vi "Get PIM System Directory.vi"(7 "Relative Path":path, 11 "Directory":T1(ring)) -> (3 "PIM Path":path)   [LabVIEW 2011]
uses:
  <vilib>/Utility/sysdir.llb/System Directory Type.ctl
panel:
  in  "Base Directory (Kaelus)":enum16{"Kaelus", "Summitek"}(ring)
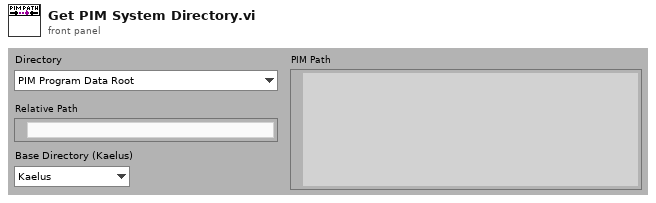
[diagram p1: front panel]
types:
  T1 = enum16{"PIM Program Data Root", "Instrument Calibration Files", "Instrument Configuration Files", "User Data", "User Configurations", "SI-90 Saved Calibrations"}
  T2 = typedef "System Directory Type.ctl" = i32
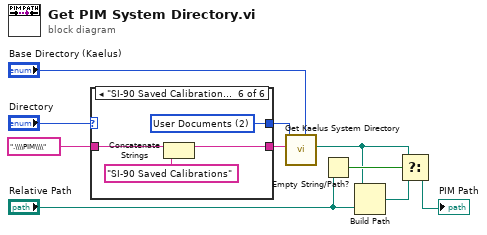
[diagram p0: block diagram]
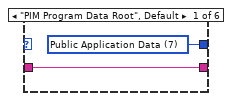
[diagram p2: hidden frame]
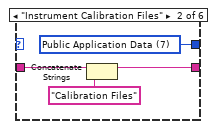
[diagram p3: hidden frame]
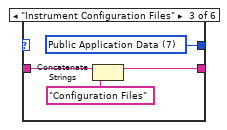
[diagram p4: hidden frame]
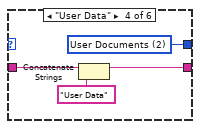
[diagram p5: hidden frame]
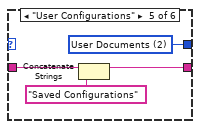
[diagram p6: hidden frame]
diagram:
  n1 = case shown="\"SI-90 Saved Calibrations\"" "Directory" {
    tunnel: ".\\\\PIM\\\\" ("Relative Application Path") -> [w12 w16 w20 w24 w28 w32]
    tunnel: [w12 w14 w18 w22 w26 w30] -> w8
    tunnel: [w11 w13 w17 w21 w25 w29] -> w2
    frame "PIM Program Data Root", Default {
      w11 = T2 7 items=["User Home", "User Desktop", "User Documents", "User Application Data", "User Preferences", "User Temporary", "Public Documents", "Public Application Data", "Public Preferences", "System Core Libraries", "System Installed Libraries", "Application Files", "Boot Volume Root"] ("Directory Type (Public App Data)")
    }
    frame "Instrument Calibration Files" {
      w13 = T2 7 items=["User Home", "User Desktop", "User Documents", "User Application Data", "User Preferences", "User Temporary", "Public Documents", "Public Application Data", "Public Preferences", "System Core Libraries", "System Installed Libraries", "Application Files", "Boot Volume Root"] ("Directory Type (Public App Data)")
      n2 = Concatenate Strings(w16, "Calibration Files" ("Relative Application Path")) -> (w14:string)
    }
    frame "Instrument Configuration Files" {
      w17 = T2 7 items=["User Home", "User Desktop", "User Documents", "User Application Data", "User Preferences", "User Temporary", "Public Documents", "Public Application Data", "Public Preferences", "System Core Libraries", "System Installed Libraries", "Application Files", "Boot Volume Root"] ("Directory Type (Public App Data)")
      n3 = Concatenate Strings(w20, "Configuration Files" ("Relative Application Path")) -> (w18:string)
    }
    frame "User Data" {
      w21 = T2 2 items=["User Home", "User Desktop", "User Documents", "User Application Data", "User Preferences", "User Temporary", "Public Documents", "Public Application Data", "Public Preferences", "System Core Libraries", "System Installed Libraries", "Application Files", "Boot Volume Root"] ("Directory Type (Public App Data)")
      n4 = Concatenate Strings(w24, "User Data" ("Relative Application Path")) -> (w22:string)
    }
    frame "User Configurations" {
      w25 = T2 2 items=["User Home", "User Desktop", "User Documents", "User Application Data", "User Preferences", "User Temporary", "Public Documents", "Public Application Data", "Public Preferences", "System Core Libraries", "System Installed Libraries", "Application Files", "Boot Volume Root"] ("Directory Type (Public App Data)")
      n5 = Concatenate Strings(w28, "Saved Configurations" ("Relative Application Path")) -> (w26:string)
    }
    frame "SI-90 Saved Calibrations" {
      w29 = T2 2 items=["User Home", "User Desktop", "User Documents", "User Application Data", "User Preferences", "User Temporary", "Public Documents", "Public Application Data", "Public Preferences", "System Core Libraries", "System Installed Libraries", "Application Files", "Boot Volume Root"] ("Directory Type (Public App Data)")
      n6 = Concatenate Strings(w32, "SI-90 Saved Calibrations" ("Relative Application Path")) -> (w30:string)
    }
  }
  n7 = call "Get Kaelus System Directory.vi"("Base Directory (Kaelus)"="Base Directory (Kaelus)", "Relative Directory Path (Directory only please)"=w8, "Directory Type (Public App Data)"=w2) -> ("Summitek ProgramData + Relative"=w5:path)  [unwired: 8 in]
  n8 = Empty String/Path?(string/path="Relative Path") -> (empty?=w6:bool)
  n9 = Build Path(base path=w5, name or relative path="Relative Path") -> (appended path=w4:path)
  n10 = Select(t=w5, s=w6, f=w4) -> (s? t:f=→"PIM Path":path)
